vi "Finish.vi"   [LabVIEW 2017]
doc: "This VI is called just before exiting. It is expected to close I/O refnum, save collected data, etc."
uses:
  <vilib>/Rock Robotics/WPI/Utilities/WPI_GetSetVariantRefNum.vi
types:
  T1 = typedef "WPI_MotorControlDeviceRef.ctl" = cluster{"DeviceStatus":errorcluster, "Type":T2, "PWM":cluster{"PWM Channel":T3, "DeadBand":T4}, "CAN":cluster{"Device Number":u8, "SetOutput VI Ref":variant, "GetOutput VI Ref":variant, "Enable VI Ref":variant, "Disable VI Ref":variant, "Data":variant}, "Invert":bool, "DIO PWM":cluster{"PWM \"Enable\" Channel":T3, "DIOChannel":T5, "PWM Rate":dbl}}
  T2 = typedef "WPI_MotorControlType.ctl" = enum16{"PWM", "CAN", "DIO PWM"}
  T3 = typedef "FPGA_DIOPWMChannel.ctl" = enum8{"PWM 0", "PWM 1", "PWM 2", "PWM 3", "PWM 4", "PWM 5", "PWM 6", "PWM 7", "PWM 8", "PWM 9", "PWM MXP 0", "PWM MXP 1", "PWM MXP 2", "PWM MXP 3", "PWM MXP 4", "PWM MXP 5", "PWM MXP 6", "PWM MXP 7", "PWM MXP 8", "PWM MXP 9", "Invalid"}
  T4 = typedef "WPI_PWMDeadband.ctl" = cluster{"Name":string, "maxPositivePwm":i32, "minPositivePwm":i32, "centerPwm":i32, "maxNegativePwm":i32, "minNegativePwm":i32, "angularRange":u16}
  T5 = typedef "FPGA_DIOChannel.ctl" = enum8{"DIO 0", "DIO 1", "DIO 2", "DIO 3", "DIO 4", "DIO 5", "DIO 6", "DIO 7", "DIO 8", "DIO 9", "DIO MXP 0", "DIO MXP 1", "DIO MXP 2", "DIO MXP 3", "DIO MXP 4", "DIO MXP 5", "DIO MXP 6", "DIO MXP 7", "DIO MXP 8", "DIO MXP 9", "DIO MXP 10", "DIO MXP 11", "DIO MXP 12", "DIO MXP 13", "DIO MXP 14", "DIO MXP 15", "SPI Port CS1", "SPI Port CS2", "SPI Port CS3", "SPI Port MISO", "SPI Port MOSI", "Invalid"}
  T6 = typedef "WPI_EncoderDevRef.ctl" = cluster{"DevStatus":errorcluster, "EncoderIndex":T7, "CounterIndex":T8, "DistancePerCount":dbl, "Decoding Type":T9}
  T7 = typedef "FPGA_EncoderIdx.ctl" = enum8{"Enc 0", "Enc 1", "Enc 2", "Enc 3", "Enc 4", "Enc 5", "Enc 6", "Enc 7", "Invalid"}
  T8 = typedef "FPGA_CounterCtrSystemIndex.ctl" = enum8{"Ctr 0", "Ctr 1", "Ctr 2", "Ctr 3", "Ctr 4", "Ctr 5", "Ctr 6", "Ctr 7", "Invalid"}
  T9 = typedef "WPI_EncoderType.ctl" = enum16{"1x", "2x", "4x"}
  T10 = typedef "WPI_JoystickDevRef.ctl" = cluster{"Device":T11}
  T11 = typedef "WPI_JoystickDeviceEnum.ctl" = enum16{"USB 0", "USB 1", "USB 2", "USB 3", "USB 4", "USB 5"}
  T12 = typedef "WPI_RobotDriveDevRef.ctl" = cluster{"DevStatus":errorcluster, "Motors[]":T1[], "Square Inputs":bool, "Max Output":dbl}
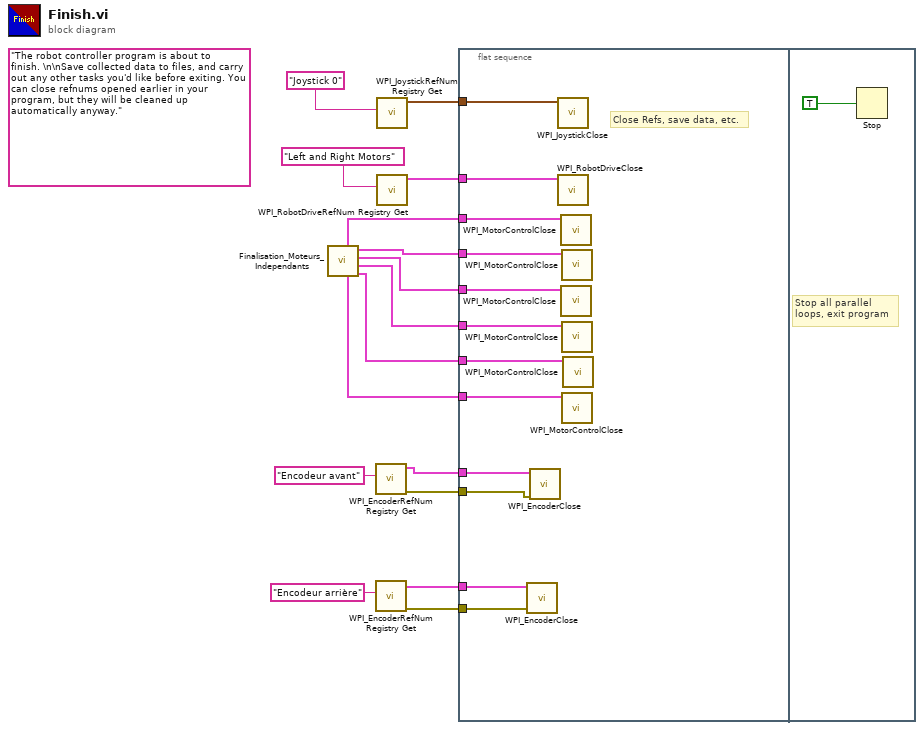
[diagram p0: block diagram]
diagram:
  (unwired) "The robot controller program is about to finish. \n\nSave collected data to files, and carry out any other tasks you'd like before exiting. You can close refnums opened earlier in your program, but they will be cleaned up automatically anyway."
  n1 = call "Finalisation_Moteurs_Independants.vi"() -> ("MotorControlDevRef 5"=w8:T1, "MotorControlDevRef 4"=w9:T1, "MotorControlDevRef 3"=w10:T1, "MotorControlDevRef 2"=w11:T1, "MotorControlDevRef 6"=w7:T1, "MotorControlDevRef"=w12:T1)  [unwired: 6 in]
  n2 = call <vilib>:"WPI_EncoderRefNum Registry Get.vi"("refnum name"="Encodeur avant") -> ("error out"=w3:errorcluster, "EncoderDevRef"=w4:T6)  [unwired: 9 in]
  n3 = call <vilib>:"WPI_EncoderRefNum Registry Get.vi"("refnum name"="Encodeur arrière") -> ("error out"=w1:errorcluster, "EncoderDevRef"=w2:T6)  [unwired: 9 in]
  n4 = call <vilib>:"WPI_JoystickRefNum Registry Get.vi"("refnum name"="Joystick 0") -> ("JoystickDevRef"=w13:T10)  [unwired: 1 in, 9 out]
  n5 = call <vilib>:"WPI_RobotDriveRefNum Registry Get.vi"("refnum name"="Left and Right Motors") -> ("RobotDriveDevRef"=w14:T12)  [unwired: 1 in, 9 out]
  n6 = flat-sequence {
    tunnel: w14 -> [w28]
    tunnel: w13 -> [w27]
    tunnel: w12 -> [w26]
    tunnel: w11 -> [w25]
    tunnel: w10 -> [w24]
    tunnel: w9 -> [w23]
    tunnel: w8 -> [w22]
    tunnel: w7 -> [w21]
    tunnel: w4 -> [w20]
    tunnel: w3 -> [w19]
    tunnel: w2 -> [w18]
    tunnel: w1 -> [w17]
    frame #0 {
      # "Close Refs, save data, etc."
      n7 = call <vilib>:"WPI_EncoderClose.vi"("error in (no error)"=w17, "EncoderDevRef"=w18) -> ()  [unwired: 9 in, 1 out]
      n8 = call <vilib>:"WPI_EncoderClose.vi"("error in (no error)"=w19, "EncoderDevRef"=w20) -> ()  [unwired: 9 in, 1 out]
      n9 = call <vilib>:"WPI_JoystickClose.vi"("JoystickDevRef"=w27) -> ()  [unwired: 11 out]
      n10 = call <vilib>:"WPI_RobotDriveClose.vi"("RobotDriveDevRef"=w28) -> ()  [unwired: 1 in, 10 out]
      n11 = call <vilib>:"WPI_MotorControlClose.vi"("MotorControlDevRef"=w26) -> ()  [unwired: 10 in, 1 out]
      n12 = call <vilib>:"WPI_MotorControlClose.vi"("MotorControlDevRef"=w24) -> ()  [unwired: 10 in, 1 out]
      n13 = call <vilib>:"WPI_MotorControlClose.vi"("MotorControlDevRef"=w25) -> ()  [unwired: 10 in, 1 out]
      n14 = call <vilib>:"WPI_MotorControlClose.vi"("MotorControlDevRef"=w23) -> ()  [unwired: 10 in, 1 out]
      n15 = call <vilib>:"WPI_MotorControlClose.vi"("MotorControlDevRef"=w21) -> ()  [unwired: 10 in, 1 out]
      n16 = call <vilib>:"WPI_MotorControlClose.vi"("MotorControlDevRef"=w22) -> ()  [unwired: 10 in, 1 out]
    }
    frame #1 {
      # "Stop all parallel\nloops, exit program"
      n17 = Stop(stop? (T)=TRUE ("Quit")) -> ()
    }
  }
